vi "get case names to array constant.vi"() -> ()   [LabVIEW 2010]
doc: "This VI demonstates how to open a reference to other open VIs and perform VI scripting actions on them."
panel:
  out "Frame Names":string[](array[string])
  out "Panel or Diagram":enum32{"Front Panel", "Block Diagram"}(ring)
  out "Objects":i32 caption="Number of Selected Objects"
  out "Types":string[](array[string]) caption="Selected Object Types"
  out "Selected VI":string
  in  "Stop":bool
  # "This VI demonstates how to open a reference to VIs that the user is interacting with and perform scripting actions on them.\n1. Run this VI\n2. Select or open any VI (for example, Demo VI is open when this VI runs).\nYou will see its name in the \"Selected VI\" control.\n3. Select objects on the other VI (either on the block diagram or front panel)\nThe types of the selected objects will be displayed in \"Selected Object Types\"\n\nSee the block diagram on code details"
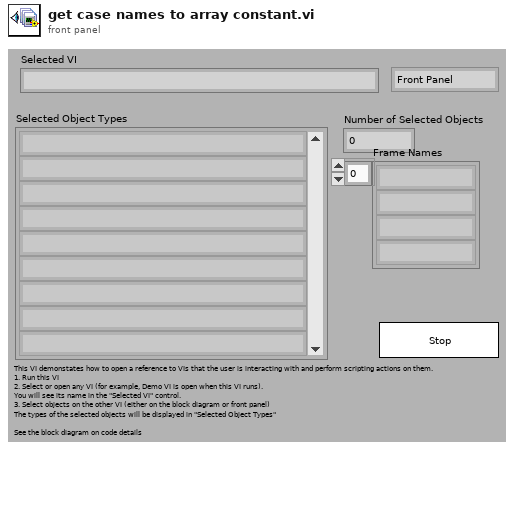
[diagram p1: front panel]
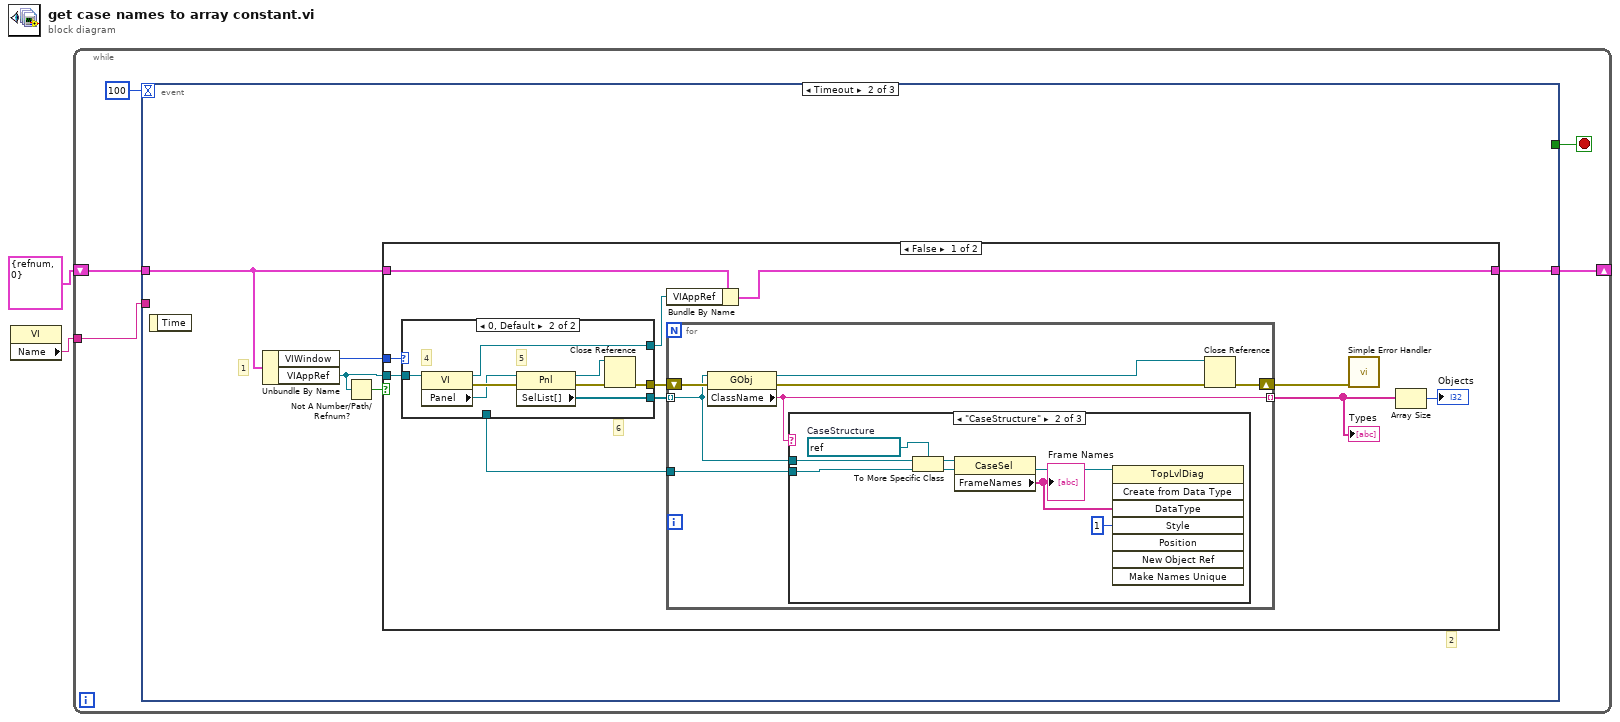
[diagram p0: block diagram]
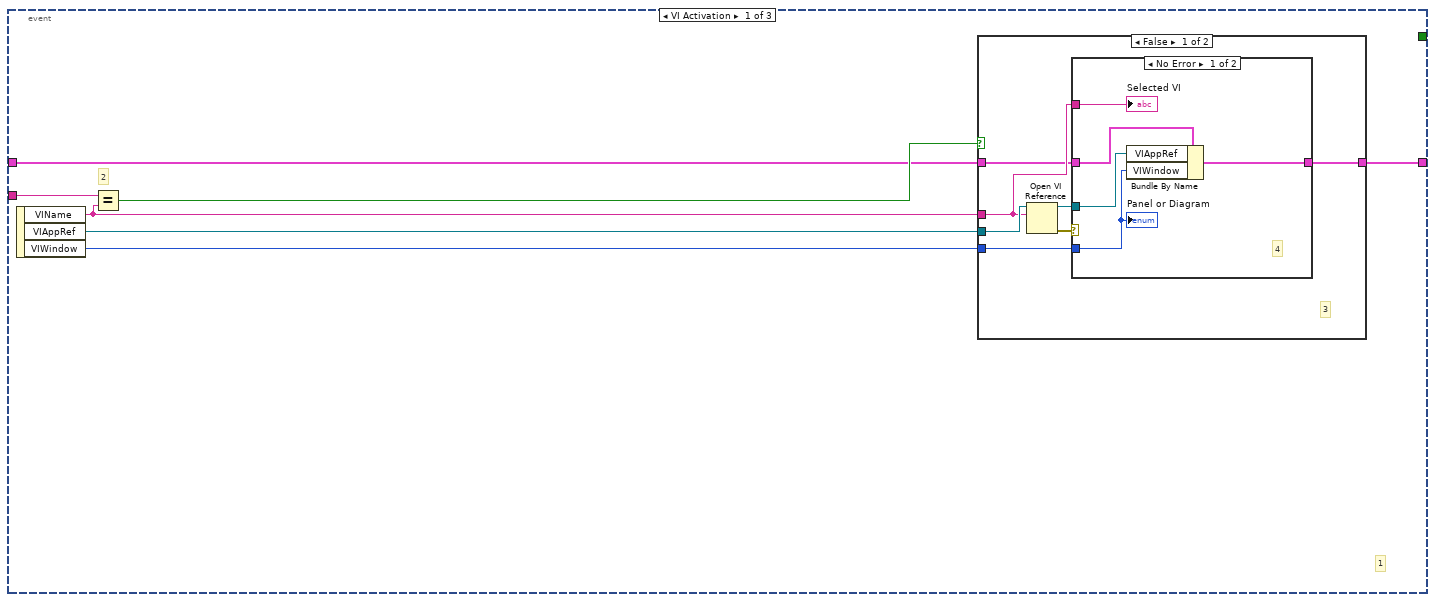
[diagram p2: hidden frame]
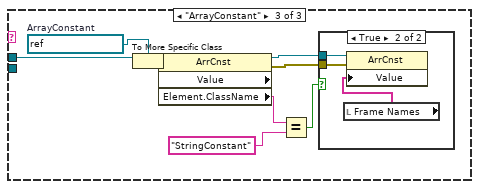
[diagram p6: hidden frame]
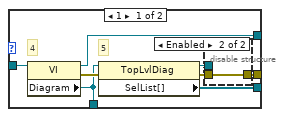
[diagram p8: hidden frame]
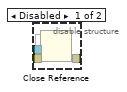
[diagram p9: hidden frame]
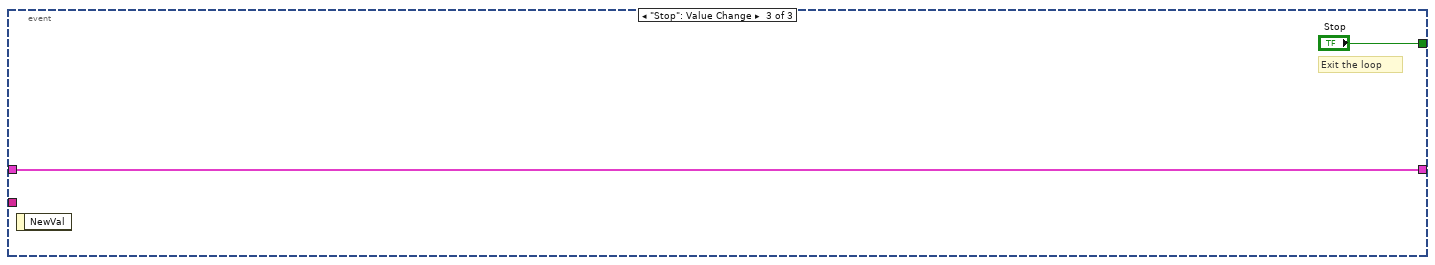
[diagram p11: hidden frame]
diagram:
  n1 = property class="VI"() -> ("Name"=w1:string)  [unwired: 2 in, 2 out]
  n2 = while {
    tunnel: w1 -> [w6]
    shift-right: [w5] -> _
    shift-left: cluster{"VIAppRef":refnum<vi>, "VIWindow":i32} {"VIAppRef"=refnum, "VIWindow"=0} -> [w4]
    stop <- w7 stop-if-true
    n3 = event shown="[1] Timeout" {
      selector: _ -> [_ _ _]
      dyn-events: _ -> [_ _ _]
      timeout: 100 -> [_ _ _]
      tunnel: [_ _ "Stop"] -> w7
      tunnel: w6 -> [w13 _ _]
      tunnel: [w9 w31 w90] -> w5
      tunnel: w4 -> [w12 w32 w90]
      event VI Activation {
        # "2"
        # "1"
        n4 = event-data() -> ("VIName"=w10:string, "VIAppRef"=w11:refnum<vi>, "VIWindow"=w8:i32)  [unwired: 1 out]
        n5 = Equal?(x=w13, y=w10) -> (x = y?=w14:bool)
        n6 = case shown="False" w14 {
          tunnel: [w16 w28] -> w9
          tunnel: w12 -> [w17 w28]
          tunnel: w10 -> [w19 _]
          tunnel: w11 -> [w21 _]
          tunnel: w8 -> [w18 _]
          frame False {
            # "3"
            n7 = Open VI Reference(application reference (local)=w21, vi path=w19) -> (vi reference=w15:refnum<vi>, error out=w20:errorcluster)  [unwired: 4 in]
            n8 = case shown="No Error" w20 {
              tunnel: w19 -> [w26 _]
              tunnel: w18 -> [w22 _]
              tunnel: w17 -> [w25 w27]
              tunnel: [w23 w27] -> w16
              tunnel: w15 -> [w24 _]
              frame No Error {
                # "4"
                n9 = Bundle By Name(cluster=w25, "VIAppRef"=w24, "VIWindow"=w22) -> (w23:cluster{"VIAppRef":refnum<vi>, "VIWindow":i32})
                "Selected VI" <- w26
                "Panel or Diagram" <- w22
              }
              frame Error {
              }
            }
          }
          frame True {
          }
        }
      }
      event Timeout {
        # "2"
        # "1"
        n10 = event-data() -> ()  [unwired: 2 out]
        n11 = Unbundle By Name(w32) -> ("VIWindow"=w30:i32, "VIAppRef"=w29:refnum<vi>)
        n12 = Not A Number/Path/Refnum?(number/path/refnum=w29) -> (NaN/Path/Refnum?=w33:bool)
        n13 = case shown="False" w33 {
          tunnel: w30 -> [w44 _]
          tunnel: w29 -> [w39 _]
          tunnel: w32 -> [w36 w89]
          tunnel: [w35 w89] -> w31
          frame False {
            # "6"
            n14 = case shown="0, Default" w44 {
              tunnel: [w75 w87] -> w43
              tunnel: [w72 w84] -> w42
              tunnel: [w74 w86] -> w37
              tunnel: w39 -> [w70 w82]
              tunnel: [w69 _] -> w34
              frame 1 {
                # "5"
                # "4"
                n15 = property class="VI"(reference=w70) -> (reference out=w74:refnum<vi>, error out=w76:errorcluster, "Diagram"=w69:refnum<vi>)  [unwired: 1 in]
                n16 = property class="TopLvlDiag"(reference=w69, error in=w76) -> (reference out=w71:refnum<vi>, error out=w73:errorcluster, "SelList[]"=w75:refnum<vi>[])
                n17 = disable-structure shown="Enabled" {
                  disable-tunnel: w73 -> [w79 w80]
                  disable-tunnel: [w78 w80] -> w72
                  disable-tunnel: w71 -> [w77 _]
                  frame Disabled {
                    n18 = Close Reference(reference=w77, error in (no error)=w79) -> (error out=w78:errorcluster)
                  }
                  frame Enabled {
                  }
                }
              }
              frame 0, Default {
                # "5"
                # "4"
                n19 = property class="VI"(reference=w82) -> (reference out=w86:refnum<vi>, error out=w88:errorcluster, "Panel"=w81:refnum<vi>)  [unwired: 1 in]
                n20 = property class="Pnl"(reference=w81, error in=w88) -> (reference out=w83:refnum<vi>, error out=w85:errorcluster, "SelList[]"=w87:refnum<vi>[])
                n21 = Close Reference(reference=w83, error in (no error)=w85) -> (error out=w84:errorcluster)
              }
            }
            n22 = Bundle By Name(cluster=w36, "VIAppRef"=w37) -> (w35:cluster{"VIAppRef":refnum<vi>, "VIWindow":i32})
            n23 = for {
              tunnel: w43 -> [w47] mode=indexing
              tunnel: [w46] -> w40 mode=indexing
              shift-right: [w49] -> w38
              shift-left: w42 -> [w51]
              tunnel: w34 -> [w45]
              n24 = property class="GObj"(reference=w47, error in=w51) -> (reference out=w48:refnum<vi>, error out=w50:errorcluster, "ClassName"=w46:string)
              n25 = case shown="\"CaseStructure\"" w46 {
                tunnel: w47 -> [_ w57 w65]
                tunnel: w45 -> [_ w54 _]
                frame "False", Default {
                }
                frame "CaseStructure" {
                  w56 = refnum<vi> refnum  # CaseStructure
                  n26 = To More Specific Class(target class=w56, reference=w57) -> (specific class reference=w55:refnum<vi>)  [unwired: 1 in, 1 out]
                  n27 = property class="CaseSel"(reference=w55) -> ("FrameNames"=w53:string[])  [unwired: 1 in, 2 out]
                  "Frame Names" <- w53
                  n28 = invoke class="TopLvlDiag" method="Create from Data Type"(reference=w54, "DataType"=w53, "Style"=1) -> ()  [unwired: 5 in, 8 out]
                }
                frame "ArrayConstant" {
                  w64 = refnum<vi> refnum  # ArrayConstant
                  n29 = To More Specific Class(target class=w64, reference=w65) -> (specific class reference=w63:refnum<vi>)  [unwired: 1 in, 1 out]
                  n30 = property class="ArrCnst" props=["Value", "Element", "ClassName"](reference=w63) -> (reference out=w60:refnum<vi>, error out=w59:errorcluster, "Element.ClassName"=w62:string)  [unwired: 1 in, 1 out]
                  n31 = Equal?(x=w62, y="StringConstant" ("Element.Class Name")) -> (x = y?=w58:bool)
                  n32 = case shown="True" w58 {
                    tunnel: w60 -> [_ w68]
                    tunnel: w59 -> [_ w67]
                    frame False {
                    }
                    frame True {
                      n33 = local read "Frame Names"() -> (w66:string[])
                      n34 = property class="ArrCnst"(reference=w68, error in=w67, "Value"=w66) -> ()  [unwired: 2 out]
                    }
                  }
                }
              }
              n35 = Close Reference(reference=w48, error in (no error)=w50) -> (error out=w49:errorcluster)
            }
            "Types" <- w40
            n36 = call <vilib>:"Simple Error Handler.vi"("error in (no error)"=w38) -> ()  [unwired: 4 in, 5 out]
            n37 = Array Size(array=w40) -> (size(s)=→"Objects":i32)
          }
          frame True {
          }
        }
      }
      event "Stop": Value Change {
        # "Exit the loop"
        n38 = event-data() -> ()  [unwired: 2 out]
      }
    }
  }
